vi "DO CO.vi"   [LabVIEW 2013]
uses:
  <vilib>/DAQmx/create/channels.llb/DAQmx Create Channel (CO-Pulse Generation-Frequency).vi
  <vilib>/DAQmx/configure/timing.llb/DAQmx Timing (Implicit).vi
  <resource>/objmgr/daqmx.rc
  <vilib>/DAQmx/configure/timing.llb/DAQmx Timing (Sample Clock).vi
  <vilib>/DAQmx/create/channels.llb/DAQmx Create Channel (AO-Voltage-Basic).vi
  <vilib>/DAQmx/write.llb/DAQmx Write (Analog Wfm 1Chan NSamp).vi
  <vilib>/measure/NI_MABase.lvlib
  <vilib>/DAQmx/configure/trigger.llb/DAQmx Start Trigger (Analog Edge).vi
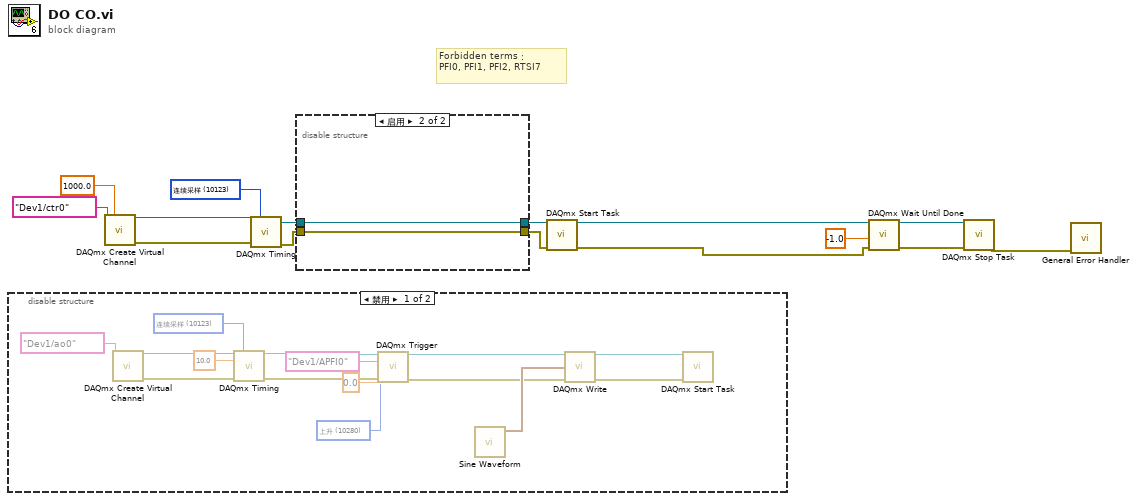
[diagram p0: block diagram]
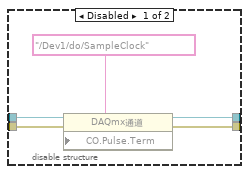
[diagram p2: hidden frame]
diagram:
  w1 = 10123 items=["有限采样"=10178, "连续采样"=10123, "硬件定时单点"=12522] ("sample mode")
  # "Forbidden terms：\nPFI0, PFI1, PFI2, RTSI7"
  n1 = disable-structure shown="禁用" {
    frame Disabled {
      w17 = 10280 items=["上升"=10280, "下降"=10171] ("slope")
      w28 = 10123 items=["有限采样"=10178, "连续采样"=10123, "硬件定时单点"=12522] ("sample mode")
      n2 = call-poly <vilib>:"DAQmx Create Virtual Channel.vi"("physical channels"=tag "Dev1/ao0") -> ("task out"=w31:refnum<k21>, "error out"=w30:errorcluster)  [unwired: 13 in]
      n3 = call-poly <vilib>:"DAQmx Timing.vi"("task/channels in"=w31, "sample mode"=w28, "rate"=10.0, "error in"=w30) -> ("task out"=w23:refnum<k21>, "source"=w16:tag, "error out"=w21:errorcluster)  [unwired: 9 in]
      n4 = call-poly <vilib>:"DAQmx Trigger.vi"("task/channels in"=w23, "source"="Dev1/APFI0", "slope"=w17, "level"=0.0, "error in"=w21) -> ("task out"=w22:refnum<k21>, "error out"=w20:errorcluster)  [unwired: 9 in]
      n5 = call <vilib>:"Sine Waveform.vi"() -> ("signal out"=w24:waveform(dbl))  [unwired: 10 in, 1 out]
      n6 = call-poly <vilib>:"DAQmx Write.vi"("task/channels in"=w22, "data"=w24, "error in"=w20) -> ("task out"=w27:refnum<k21>, "error out"=w26:errorcluster)  [unwired: 10 in, 1 out]
      n7 = call <vilib>:"DAQmx Start Task.vi"("task/channels in"=w27, "error in"=w26) -> ()  [unwired: 12 in, 2 out]
    }
    frame Enabled {
    }
  }
  n8 = call-poly <vilib>:"DAQmx Create Virtual Channel.vi"("frequency"=1000.0, "counter"=tag "Dev1/ctr0") -> ("task out"=w15:refnum<k21>, "error out"=w14:errorcluster)  [unwired: 12 in]
  n9 = call-poly <vilib>:"DAQmx Timing.vi"("task/channels in"=w15, "sample mode"=w1, "error in"=w14) -> ("task out"=w12:refnum<k21>, "error out"=w11:errorcluster)  [unwired: 11 in]
  n10 = disable-structure shown="启用" {
    disable-tunnel: w12 -> [w36 w38]
    disable-tunnel: w11 -> [w35 w37]
    disable-tunnel: [w34 w38] -> w10
    disable-tunnel: [w33 w37] -> w9
    frame Disabled {
      n11 = property class="DAQmx通道"(reference=w36, error in=w35, "CO.Pulse.Term"=tag "/Dev1/do/SampleClock") -> (reference out=w34:refnum<k21>, error out=w33:errorcluster)
    }
    frame Enabled {
    }
  }
  n12 = call <vilib>:"DAQmx Start Task.vi"("task/channels in"=w10, "error in"=w9) -> ("task out"=w7:refnum<k21>, "error out"=w2:errorcluster)  [unwired: 12 in]
  n13 = call <vilib>:"DAQmx Wait Until Done.vi"("task/channels in"=w7, "timeout (sec)"=-1.0, "error in"=w2) -> ("task out"=w6:refnum<k21>, "error out"=w5:errorcluster)  [unwired: 11 in]
  n14 = call <vilib>:"DAQmx Stop Task.vi"("task/channels in"=w6, "error in"=w5) -> ("error out"=w3:errorcluster)  [unwired: 12 in, 1 out]
  n15 = call <vilib>:"General Error Handler.vi"("error in (no error)"=w3) -> ()  [unwired: 10 in, 5 out]
